vi "_USB_CAN_DEBUG_LOG_1.vi"(10 "Info":string, 11 "TIME":timestamp) -> ()   [LabVIEW 2011]
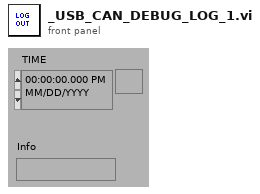
[diagram p1: front panel]
types:
  T1 = enum16{"open", "replace", "create", "open or create", "replace or create", "replace or create with confirmation"}
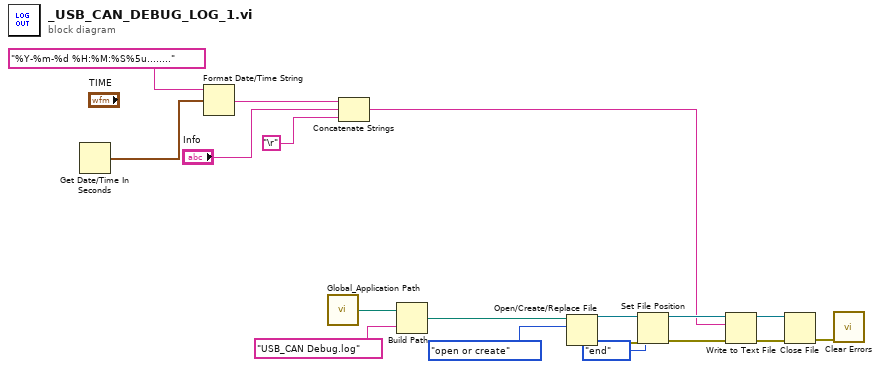
[diagram p0: block diagram]
diagram:
  n1 = Get Date/Time In Seconds() -> (seconds since 1Jan1904=w1:timestamp)
  n2 = Format Date/Time String(time format string (%c)="%Y-%m-%d %H:%M:%S%5u........" ("时间格式字符串(%c)"), seconds (now)=w1) -> (date/time string=w5:string)  [unwired: 1 in]
  n3 = call "Global_Application Path.vi"() -> ("程序路径"=w7:path)  [unwired: 1 in]
  n4 = Concatenate Strings(w5, "Info", "\r") -> (w2:string)
  n5 = Build Path(base path=w7, name or relative path="USB_CAN Debug.log" ("名称或相对路径")) -> (appended path=w17:path)
  n6 = Open/Create/Replace File(file path (use dialog)=w17, operation (0:open)=T1."open or create" ("操作(0:open)")) -> (refnum out=w15:refnum<file>, error out=w14:errorcluster)  [unwired: 4 in, 1 out]
  n7 = Set File Position(refnum=w15, from (0:start)=enum16{"start", "end", "current"}."end" ("自（0:起始）"), error in=w14) -> (refnum out=w12:refnum<file>, error out=w11:errorcluster)  [unwired: 1 in]
  n8 = Write to Text File(file (use dialog)=w12, text=w2, error in=w11) -> (refnum out=w9:refnum<file>, error out=w10:errorcluster)  [unwired: 1 in, 1 out]
  n9 = Close File(refnum=w9, error in=w10) -> (error out=w8:errorcluster)  [unwired: 1 out]
  n10 = call <vilib>:"Clear Errors.vi"("error in (no error)"=w8) -> ()  [unwired: 6 in, 1 out]
